vi "Enumerate Banana Peels.vi"(11 "Platano":refnum<class "Platano.lvclass">) -> (2 "Peels":set{refnum<class "BananaPeel.lvclass">}(c389), 3 "Platano":refnum<class "Platano.lvclass">)   [LabVIEW 2021, in "Bananas.lvlib" / "Platano.lvclass"]
uses:
  Platano.lvclass
  Banana/Banana.lvclass
  BananaPeel/BananaPeel.lvclass
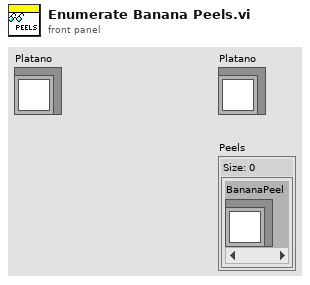
[diagram p1: front panel]
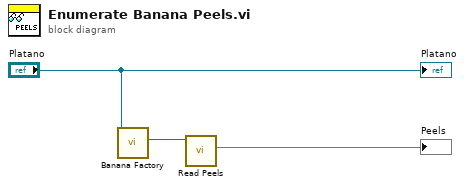
[diagram p0: block diagram]
diagram:
  n1 = call "Banana Factory.vi"("Platano"="Platano") -> ("Banana"=w1:refnum<class "Banana.lvclass">)  [unwired: 9 in, 1 out]
  n2 = call "Read Peels.vi"("Banana in"=w1) -> ("Peels"=→"Peels":set{refnum<class "BananaPeel.lvclass">})  [unwired: 8 in, 2 out]
  "Platano" <- "Platano"
